vi "Fetch PRACH IQ Constellation Trace Results.vi"(8 "error in (no error)":errorcluster, 10 "Instance (1)":T1=1, 11 "VISA resource name":refnum<visa-resource-name>) -> (0 "error out":errorcluster, 1 "Results":dbl[](array[numeric]) format="%^.3e", 2 "Reliability":i32, 3 "VISA resource name out":refnum<visa-resource-name>)   [LabVIEW 2020, in "Rohde&Schwarz CMWXP NR FR1 Measurement.lvlib"]
doc: "Returns the results in the I/Q constellation diagram. There is one pair of values per modulation symbol. The number of modulation symbols equals the number of subcarriers and depends on the preamble format. The results are returned in the following order: <Reliability>, {<IPhase>, <QPhase>}symbol 1, ..., {<IPhase>, <QPhase>}symbol n\n\nAttribute:\nRSCMWXPNRFR1M_ATTR_FETCH_PRACH_IQ_CONSTELLATION_TRACE_RESULTS\n\nRemote-control command:\nFETCh:NRSub:MEAS<i>:PRACh:TRACe:IQ?"
uses:
  <instrlib>/Rohde&Schwarz CMWXP NR FR1 Measurement/Rohde&Schwarz CMWXP NR FR1 Measurement.lvlib
  <instrlib>/Rohde&Schwarz CMWXP NR FR1 Measurement/Private/_Instance.ctl
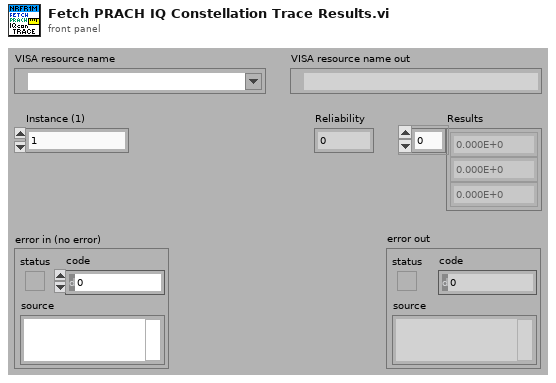
[diagram p1: front panel]
types:
  T1 = typedef "Rohde&Schwarz CMWXP NR FR1 Measurement.lvlib/_Instance.ctl" = i32
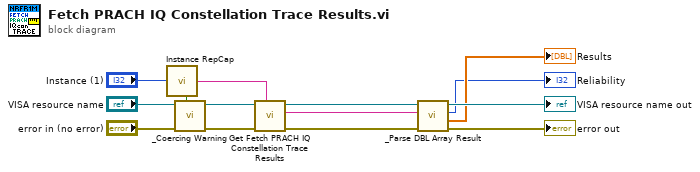
[diagram p0: block diagram]
diagram:
  n1 = call <instrlib>:"Instance RepCap.vi"("Instance In"="Instance (1)") -> ("In Range?"=w8:bool, "RepCap Identifier Out"=w9:string)  [unwired: 1 in]
  n2 = call <instrlib>:"_Coercing Warning.vi"("In Range?"=w8, "error in (no error)"="error in (no error)", "VISA resource name"="VISA resource name") -> ("error out"=w12:errorcluster, "VISA resource name out"=w11:refnum<visa-resource-name>)  [unwired: 7 in]
  n3 = call "Get Fetch PRACH IQ Constellation Trace Results"("Repeated Capabilities"=w9, "error in (no error)"=w12, "instrument handle"=w11) -> ("error out"=w7:errorcluster, "Fetch PRACH IQ Constellation Trace Results"=w1:string, "instrument handle out"=w4:refnum<visa-resource-name>)  [unwired: 6 in]
  n4 = call <instrlib>:"_Parse DBL Array Result.vi"("error in (no error)"=w7, "Input String"=w1, "VISA resource name"=w4) -> ("error out"=→"error out":errorcluster, "Results"=→"Results":dbl[], "Reliability"=→"Reliability":i32, "VISA resource name out"=→"VISA resource name out":refnum<visa-resource-name>)  [unwired: 5 in]
